vi "gentec-SOLO-PE.set Scale.vi"(8 "error in (no error)":errorcluster, 10 "Scale":T1 items=["Auto", "1 pJ", "3 pJ", "10 pJ", "30 pJ", "100 pJ", "300 pJ", "1 nJ", "3 nJ", "10 nJ", "30 nJ", "100 nJ", "300 nJ", "1 uJ", "3 uJ", "10 uJ", "30 uJ", "100 uJ", "300 uJ", "1 mJ", "3 mJ", "10 mJ", "30 mJ", "100 mJ", "300 mJ", "1 J", "3 J", "10 J", "30 J", "100 J", "300 J", "1 kJ", "3 kJ", "10 kJ", "30 kJ", "100 kJ", "300 kJ", "1 MJ", "3 MJ", "10 MJ", "30 MJ", "100 MJ", "300 MJ"], 11 "VISA Refnum in":refnum<visa-resource-name>) -> (0 "error out":errorcluster, 1 "Acknoledged?":bool, 2 "Error":string, 3 "VISA Refnum out":refnum<visa-resource-name>, 4 "Timeout":bool)   [LabVIEW 2014, in "gentec-SOLO-PE - Driver.lvlib"]
doc: "Sets the Scaling; 0 is auto."
uses:
  gentec-SOLO-PE - Driver.lvlib
  Type Defs/gentec-SOLO-PE.Scale.ctl
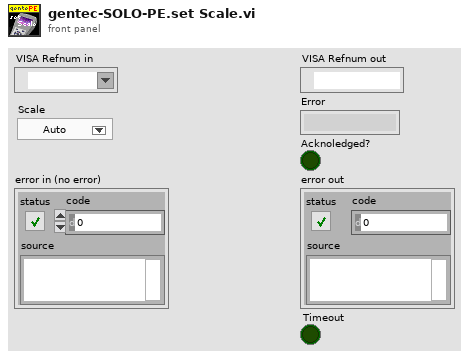
[diagram p1: front panel]
types:
  T1 = typedef "gentec-SOLO-PE - Driver.lvlib/gentec-SOLO-PE.Scale.ctl" = u32
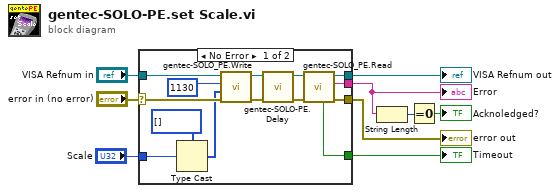
[diagram p0: block diagram]
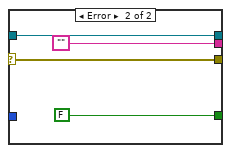
[diagram p2: hidden frame]
diagram:
  n1 = case shown="No Error" "error in (no error)" {
    selector: "error in (no error)" -> [w21 w26]
    tunnel: [w20 w26] -> w9
    tunnel: [w23 w27] -> w8
    tunnel: [w18 ""] -> w4
    tunnel: [w17 FALSE ("Timeout")] -> w7
    tunnel: "VISA Refnum in" -> [w22 w27]
    tunnel: "Scale" -> [w19 _]
    frame No Error {
      n2 = Type Cast(type=u32[] [], x=w19) -> (*(type *) &x=w12:u32[])
      n3 = call "gentec-SOLO_PE.Write.vi"("error in (no error)"=w21, "Parameters (Empty)"=w12, "Command Handle"=u16 1130, "VISA Refnum in"=w22) -> ("error out"=w16:errorcluster, "VISA Refnum out"=w15:refnum<visa-resource-name>)  [unwired: 6 in]
      n4 = call "gentec-SOLO-PE.Delay.vi"("error in (no error)"=w16, "VISA resource In"=w15) -> ("error out"=w11:errorcluster, "VISA resource Out"=w10:refnum<visa-resource-name>)  [unwired: 4 in]
      n5 = call "gentec-SOLO_PE.Read.vi"("error in (no error)"=w11, "VISA Refnum in"=w10) -> ("error out"=w20:errorcluster, "Error"=w18:string, "VISA Refnum out"=w23:refnum<visa-resource-name>, "Timeout"=w17:bool)  [unwired: 5 in, 1 out]
    }
    frame Error {
    }
  }
  "error out" <- w9
  "VISA Refnum out" <- w8
  "Error" <- w4
  "Timeout" <- w7
  n6 = String Length(string=w4) -> (length=w3:i32)
  n7 = Equal To 0?(x=w3) -> (x = 0?=→"Acknoledged?":bool)
